vi "Read configuration.vi"(8 "error in":errorcluster, 11 "GPIC ScaleAndLimit editor node in":refnum<class "GPIC ScaleAndLimit editor node.lvclass">) -> (0 "error out":errorcluster, 2 "configuration":refnum<class "NISE_CEF_serializable configuration.lvclass">, 3 "GPIC ScaleAndLimit editor node out":refnum<class "GPIC ScaleAndLimit editor node.lvclass">)   [LabVIEW 2015, in "GPIC ScaleAndLimit editor node.lvclass"]
uses:
  GPIC ScaleAndLimit editor node.lvclass
  <vilib>/NI/Configuration Framework/serializable configuration/NISE_CEF_serializable configuration.lvclass
  GPIC ScaleAndLimit editor node.lvclass/GPIC ScaleAndLimit editor node.ctl
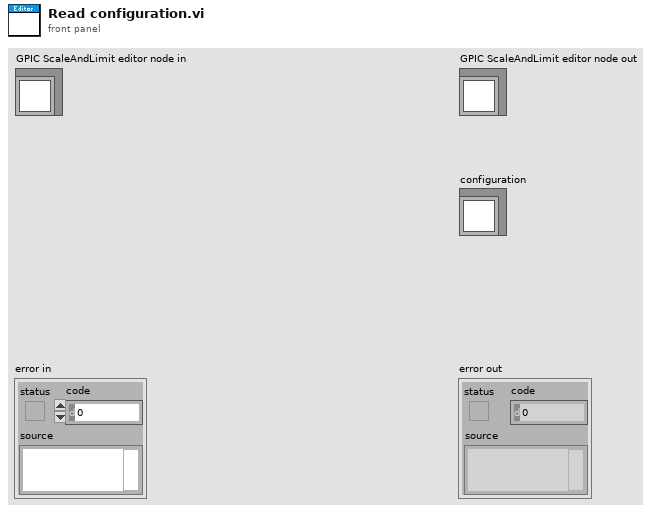
[diagram p1: front panel]
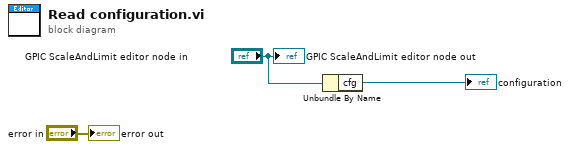
[diagram p0: block diagram]
diagram:
  n1 = Unbundle By Name("GPIC ScaleAndLimit editor node in") -> ("cfg"=→"configuration":refnum<class "GPIC ScaleAndLimit configuration.lvclass">)
  "error out" <- "error in"
  "GPIC ScaleAndLimit editor node out" <- "GPIC ScaleAndLimit editor node in"
